vi "ADC Example (B).vi"() -> ()   [LabVIEW 2011]
doc: "Control the Analog/Digital converter with constant values (basic version)."
uses:
  C:/Program Files/Metrohm Autolab/Autolab SDK 1.10/EcoChemie.Autolab.Sdk.dll
  EcoChemie.Autolab.Sdk.dll
panel:
  out "IsConnected":bool
  in  "stop":bool
  out "error out":errorcluster
  out "ADC channel 3":dbl
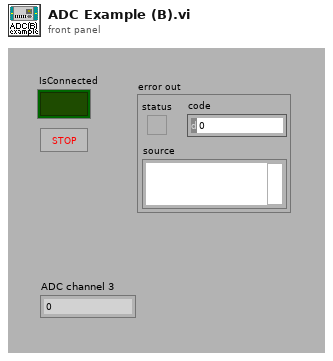
[diagram p1: front panel]
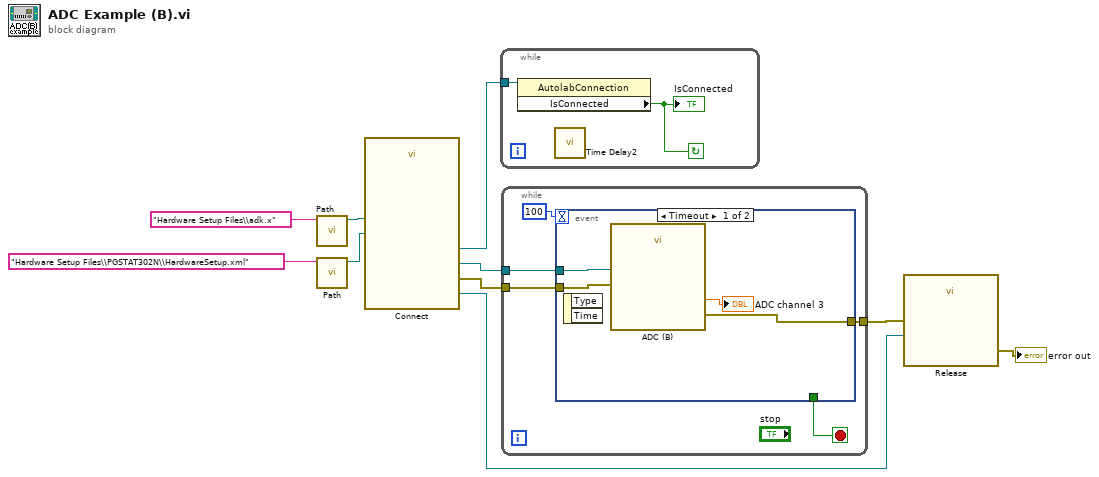
[diagram p0: block diagram]
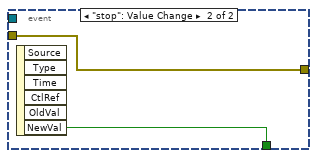
[diagram p2: hidden frame]
diagram:
  n1 = call "Path.vi"("name or relative path"="Hardware Setup Files\\adk.x") -> ("appended path"=w3:path)  [unwired: 10 in]
  n2 = call "Path.vi"("name or relative path"="Hardware Setup Files\\PGSTAT302N\\HardwareSetup.xml") -> ("appended path"=w2:path)  [unwired: 10 in]
  n3 = call "Connect.vi"("Embedded Exe File"=w3, "Hardware Setup File"=w2) -> ("Adc"=w9:refnum<k24>, "AutolabConnection"=w10:refnum<k24>, "instrument"=w7:refnum<k24>, "error out"=w8:errorcluster)  [unwired: 6 in, 4 out]
  n4 = while {
    tunnel: w10 -> [w11]
    stop <- w12 continue-if-true
    n5 = property class="AutolabConnection"(reference=w11) -> ("IsConnected"=w12:bool)  [unwired: 1 in, 2 out]
    "IsConnected" <- w12
    n6 = call "Time Delay2"() -> ()  [unwired: 11 in, 1 out]
  }
  n7 = while {
    tunnel: w8 -> [w15]
    tunnel: w9 -> [w16]
    tunnel: [w13] -> w1
    stop <- w14 stop-if-true
    n8 = event shown="[0] Timeout" {
      selector: _ -> [_ _]
      dyn-events: _ -> [_ _]
      timeout: 100 ("Numeric") -> [_ _]
      tunnel: [_ w23] -> w14
      tunnel: w16 -> [w20 _]
      tunnel: w15 -> [w19 w22]
      tunnel: [w18 w22] -> w13
      event Timeout {
        n9 = event-data() -> ()  [unwired: 1 in, 2 out]
        n10 = call "ADC (B).vi"("error in"=w19, "Adc"=w20) -> ("error out"=w18:errorcluster, "Sample"=→"ADC channel 3":dbl)  [unwired: 8 in]
      }
      event "stop": Value Change {
        n11 = event-data() -> ("NewVal"=w23:bool)  [unwired: 1 in, 5 out]
      }
    }
  }
  n12 = call "Release.vi"("error in (no error)"=w1, "Instrument"=w7) -> ("error out"=→"error out":errorcluster)  [unwired: 9 in]
